vi "Create Input Test Configuration.vi"(10 "Connection Configuration":T2={"Client?"=FALSE, "Server Certificates"={"Relative Path?"=FALSE, "Certificate Paths"=[], "Certificate Names"=[]}, "Client Certificates"={"Relative Path?"=FALSE, "Certificate Paths"=[], "Certificate Names"=[]}, "Client Configuration"={"Server Endpoint URL"="", "Security Policy"={"Message Mode"=enum."None", "Security"=enum."Basic256"}, "Username/Password"={"Username"="", "Password"=""}}, "Server Configuration"={"Server Name"="", "TCP port (49580)"="49580", "Supported Security Policies"={"None"=TRUE, "Sign with Basic128Rsa125"=FALSE, "Sign and Encrypt with Basic128Rsa125"=FALSE, "Sign with Basic256"=FALSE, "Sign and Encrypt with Basic256"=FALSE}}}) -> (0 "error out":errorcluster, 1 "Names":string[](array[string]), 2 "Items":cluster{string, "OPC UA Data Type":T3}[](array[cluster]) {"OPC UA Data Type" items=["Boolean"=1, "SByte"=2, "Byte"=3, "Int16"=4, "UInt16"=5, "Int32"=6, "UInt32"=7, "Int64"=8, "UInt64"=9, "Float"=10, "Double"=11, "String"=12, "DateTime"=13, "ByteString"=15, "Array of Boolean"=101, "Array of SByte"=102, "Array of Byte"=103, "Array of Int16"=104, "Array of UInt16"=105, "Array of Int32"=106, "Array of UInt32"=107, "Array of Int64"=108, "Array of UInt64"=109, "Array of Float"=110, "Array of Double"=111, "Array of String"=112, "Array of DateTime"=113, "Array of ByteString"=115]}, 3 "module":refnum<class "OPC UA Server configuration.lvclass">, 4 "Channels":refnum<class "TBM channel.lvclass">[](array[class]), 5 "instance identifier":string)   [LabVIEW 2013, in "OPC UA Server tests.lvlib"]
doc: "This VI creates the test configuration used in testing. BY default just creates one line with every datatype"
uses:
  OPC UA Server tests.lvlib
  module/configuration/OPC UA Server configuration.lvclass
  <vilib>/NI/Tag Bus Module Framework/channel/TBM channel.lvclass
  module/configuration/OPC UA Data Type.ctl
  <vilib>/OPCUA/server/subVI/supported security policies.ctl
  <vilib>/NI/Tag Bus Module Framework/channel/channel classification.ctl
  module/configuration/Line.ctl
  module/configuration/OPC UA Server configuration.lvclass/OPC UA Server configuration.ctl
  module/configuration/Write Connection Configuration.vi
  <vilib>/NI/Configuration Framework/serializable configuration/NISE_CEF_serializable configuration.lvclass
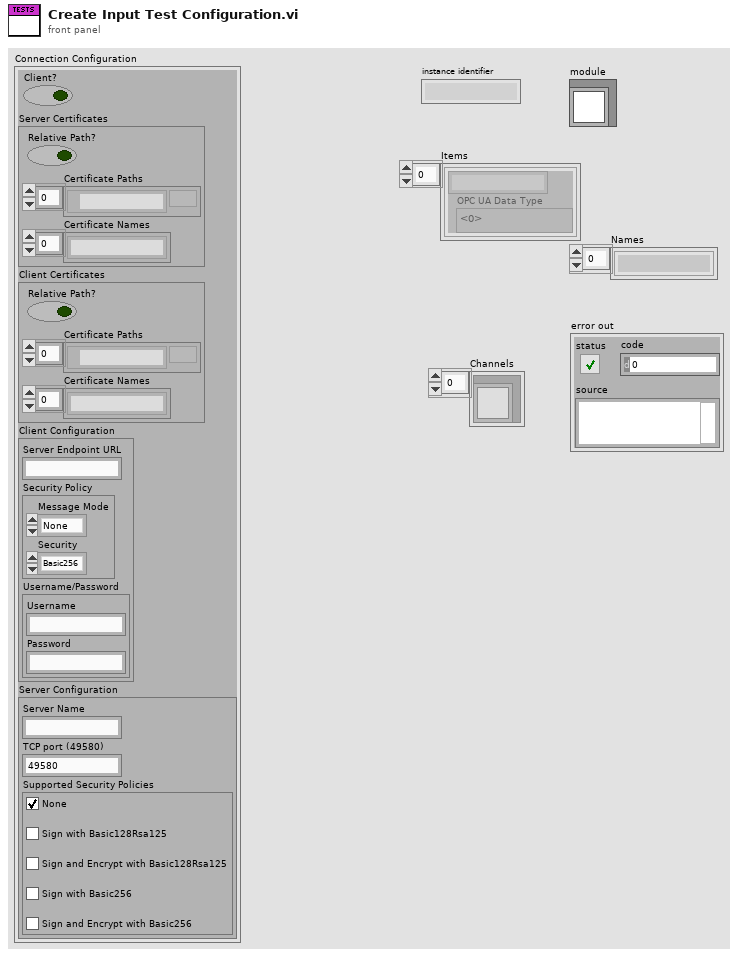
[diagram p1: front panel]
types:
  T1 = typedef "supported security policies.ctl" = cluster{"None":bool, "Sign with Basic128Rsa125":bool, "Sign and Encrypt with Basic128Rsa125":bool, "Sign with Basic256":bool, "Sign and Encrypt with Basic256":bool}
  T2 = cluster{"Client?":bool, "Server Certificates":cluster{"Relative Path?":bool, "Certificate Paths":path[], "Certificate Names":string[]}, "Client Certificates":cluster{"Relative Path?":bool, "Certificate Paths":path[], "Certificate Names":string[]}, "Client Configuration":cluster{"Server Endpoint URL":string, "Security Policy":cluster{"Message Mode":enum16{"None", "Sign", "Sign and Encrypt"}, "Security":enum16{"Basic256", "Basic128Rsa15"}}, "Username/Password":cluster{"Username":string, "Password":string}}, "Server Configuration":cluster{"Server Name":string, "TCP port (49580)":string, "Supported Security Policies":T1}}
  T3 = typedef "OPC UA Server configuration.lvclass/OPC UA Data Type.ctl" = u16
  T4 = typedef "TBM channel.lvclass/channel classification.ctl" = enum16{"input data", "output data", "processing parameter", "processing result"}
  T5 = typedef "OPC UA Server configuration.lvclass/Line.ctl" = cluster{"channel":refnum<class "TBM channel.lvclass">, "Node Path":string, "OPC UA Data Type":T3}
  T6 = typedef "tag bus.lvlib/tag descriptor.lvclass/Data Type.ctl" = enum16{"Double", "Single", "I64", "I32", "I16", "I8", "U64", "U32", "U16", "U8", "Boolean", "String", "Array of Double", "Array of Single", "Array of I64", "Array of I32", "Array of I16", "Array of I8", "Array of U64", "Array of U32", "Array of U16", "Array of U8", "Array of Boolean", "Array of String"}
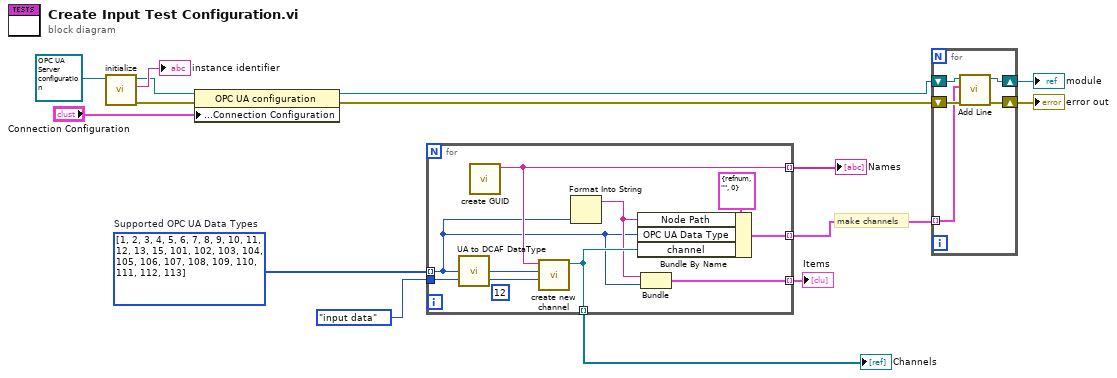
[diagram p0: block diagram]
diagram:
  w1 = T3[] [1, 2, 3, 4, 5, 6, 7, 8, 9, 10, 11, 12, 13, 15, 101, 102, 103, 104, 105, 106, 107, 108, 109, 110, 111, 112, 113] items=["Boolean"=1, "SByte"=2, "Byte"=3, "Int16"=4, "UInt16"=5, "Int32"=6, "UInt32"=7, "Int64"=8, "UInt64"=9, "Float"=10, "Double"=11, "String"=12, "DateTime"=13, "ByteString"=15, "Array of Boolean"=101, "Array of SByte"=102, "Array of Byte"=103, "Array of Int16"=104, "Array of UInt16"=105, "Array of Int32"=106, "Array of UInt32"=107, "Array of Int64"=108, "Array of UInt64"=109, "Array of Float"=110, "Array of Double"=111, "Array of String"=112, "Array of DateTime"=113, "Array of ByteString"=115]  # Supported OPC UA Data Types
  # "make channels"
  n1 = call <vilib>:"initialize.vi"("configuration in"=refnum<class "OPC UA Server configuration.lvclass"> refnum ("tag bus configurable plugin module configuration")) -> ("error out"=w13:errorcluster, "identifier"=→"instance identifier":string, "configuration out"=w10:refnum<class "OPC UA Server configuration.lvclass">)  [unwired: 8 in]
  n2 = property class="OPC UA configuration"(reference=w10, error in=w13, "Customize:Properties:Connection Configuration"="Connection Configuration") -> (reference out=w6:refnum<class "OPC UA Server configuration.lvclass">, error out=w12:errorcluster)
  n3 = for {
    tunnel: channel_classification."input data" ("channel classification") -> [w24]
    tunnel: [w21] -> w9 mode=indexing
    tunnel: w1 -> [w17] mode=indexing
    tunnel: [w23] -> w11 mode=indexing
    tunnel: [w20] -> w5 mode=indexing
    tunnel: [w16] -> w3 mode=indexing
    (unwired) 12
    n4 = call "UA to DCAF DataType.vi"("OPC UA Data Type"=w17) -> ("DCAF Datatype"=w19:T6)
    n5 = call <vilib>:"create GUID.vi"() -> ("uuid"=w23:string)  [unwired: 10 in, 1 out]
    n6 = call <vilib>:"create new channel.vi"("channel classification"=w24, "data type"=w19, "channel name"=w23) -> ("channel"=w20:refnum<class "TBM channel.lvclass">)  [unwired: 8 in]
    n7 = Format Into String(w17) -> (resulting string=w18:string)  [unwired: 3 in, 1 out]
    n8 = Bundle By Name(cluster=T5 {"channel"=refnum, "Node Path"="", "OPC UA Data Type"=0} ("Line"), "Node Path"=w18, "OPC UA Data Type"=w17, "channel"=w20) -> (w21:T5)
    n9 = Bundle(w18, "OPC UA Data Type"=w17) -> (w16:cluster{string, "OPC UA Data Type":T3})  [unwired: 1 in]
  }
  "Names" <- w11
  "Channels" <- w5
  "Items" <- w3
  n10 = for {
    tunnel: w9 -> [w25] mode=indexing
    shift-right: [w28] -> w8
    shift-left: w6 -> [w29]
    shift-right: [w26] -> w15
    shift-left: w12 -> [w27]
    n11 = call "Add Line.vi"("error in"=w27, "Line"=w25, "OPC UA configuration in"=w29) -> ("error out"=w26:errorcluster, "OPC UA configuration out"=w28:refnum<class "OPC UA Server configuration.lvclass">)  [unwired: 7 in]
  }
  "error out" <- w15
  "module" <- w8
